vi "Write QObject Class Ref.vi"(8 "error in (no error)":errorcluster, 10 "QObject Class Ref":refnum<vi>, 11 "QObject Writer in":refnum<class "QObject Writer.lvclass">) -> (0 "error out":errorcluster, 3 "QObject Writer out":refnum<class "QObject Writer.lvclass">)   [LabVIEW 2013, in "QObject Writer.lvclass"]
uses:
  QObject Writer.lvclass
  QObject Writer.lvclass/QObject Writer.ctl
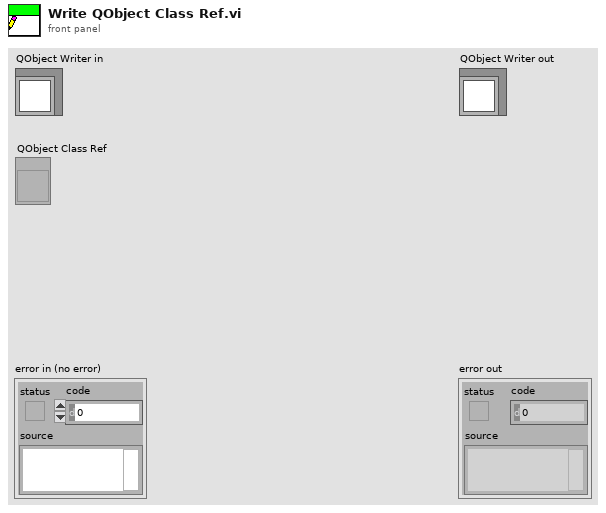
[diagram p1: front panel]
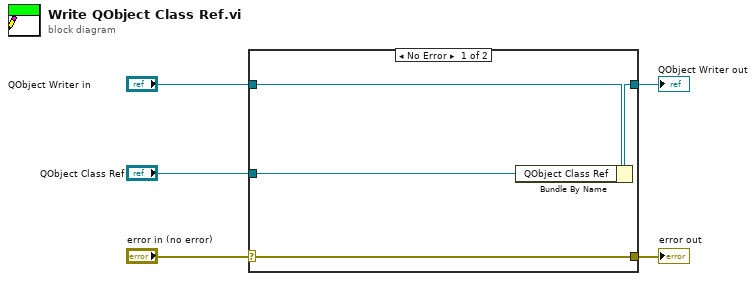
[diagram p0: block diagram]
diagram:
  n1 = case shown="No Error" "error in (no error)" {
    selector: "error in (no error)" -> [w9 w10]
    tunnel: [w9 w10] -> w4
    tunnel: [w7 w11] -> w2
    tunnel: "QObject Writer in" -> [w8 w11]
    tunnel: "QObject Class Ref" -> [w6 _]
    frame No Error {
      n2 = Bundle By Name(cluster=w8, "QObject Class Ref"=w6) -> (w7:refnum<class "QObject Writer.lvclass">)
    }
    frame Error {
    }
  }
  "error out" <- w4
  "QObject Writer out" <- w2
